vi "ActionVIOnDelete.vi"(6 "All deleted Refs":T1[](array[typedef]) format="%.0x", 8 "error in (no error)":errorcluster, 11 "Item Ref in":T1 format="%.0x") -> (0 "error out":errorcluster, 3 "Item Ref out":T1 format="%.0x")   [LabVIEW 2013, in "J1939 Addon System Explorer.lvlib"]
uses:
  J1939 Addon System Explorer.lvlib
  <vilib>/NI Veristand/Custom Device API/Custom Device Item Ref.ctl
  Shared/Types/XNET Settings.ctl
  Shared/SubVIs/Constants.vi
  <vilib>/NI Veristand/Custom Device API/Get Item Property (Variant).vi
  <vilib>/NI Veristand/Custom Device Tools/Custom Device Utility Library/NI VeriStand - Search for Item by GUID.vi
  <vilib>/NI Veristand/Custom Device Tools/Custom Device Utility Library/NI VeriStand - Search for Item by Name.vi
  Shared/J1939 Addon Shared.lvlib
  <vilib>/NI Veristand/Custom Device API/Custom Device API.lvlib
  <vilib>/NI Veristand/Custom Device Tools/Custom Device Utility Library/Custom Device Utility Library.lvlib
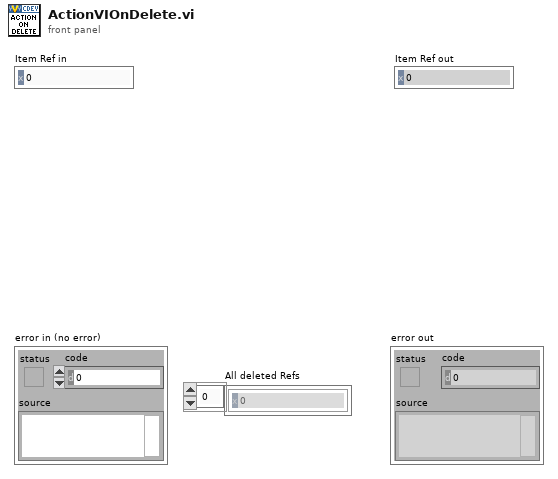
[diagram p1: front panel]
types:
  T1 = typedef "Custom Device API.lvlib/Custom Device Item Ref.ctl" = u64
  T2 = typedef "J1939 Addon Shared.lvlib/XNET Settings.ctl" = cluster{"Database":refnum<k21>, "Cluster":refnum<k21>, "Port":string, "Baud rate [Bd]":u32, "Termination":u32, "Incoming Rate":u32, "Outcoming Rate":u32, "Write Decimation":u32}
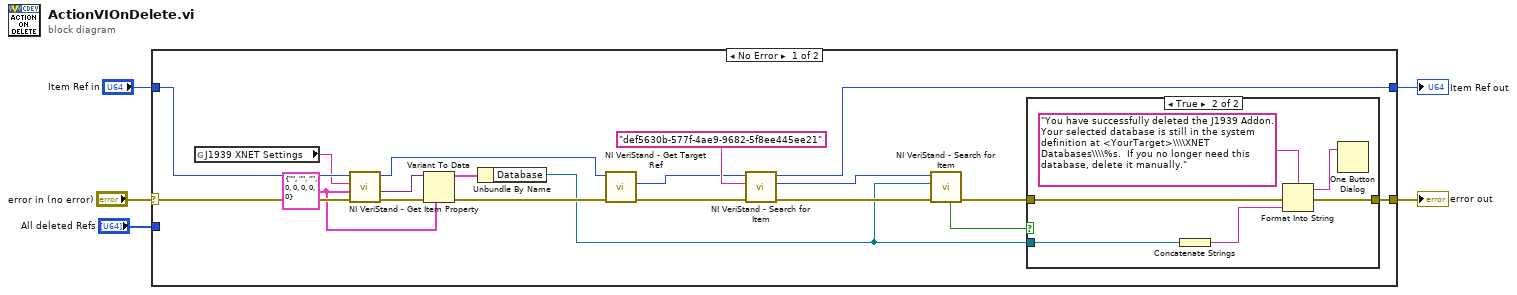
[diagram p0: block diagram]
diagram:
  n1 = case shown="No Error" "error in (no error)" {
    selector: "error in (no error)" -> [w24 w33]
    tunnel: [w22 w33] -> w4
    tunnel: "Item Ref in" -> [w23 w32]
    tunnel: [w21 w32] -> w2
    tunnel: "All deleted Refs" -> [_ _]
    frame No Error {
      w17 = T2 {"Database"="", "Cluster"="", "Port"="", "Baud rate [Bd]"=0, "Termination"=0, "Incoming Rate"=0, "Outcoming Rate"=0, "Write Decimation"=0} ("J1939 XNET Settings")
      n2 = global read "Constants.vi" "J1939 XNET Settings"() -> (w20:string)
      n3 = call-poly <vilib>:"NI VeriStand - Get Item Property.vi"("error in (no error)"=w24, "Default Value"=w17, "Property Name"=w20, "Item Ref in"=w23) -> ("error out"=w18:errorcluster, "Value"=w19:variant, "Item Ref out"=w10:T1)  [unwired: 4 in, 1 out]
      n4 = Variant To Data(error in=w18, type=w17, Variant=w19) -> (data=w16:T2, error out=w8:errorcluster)
      n5 = Unbundle By Name(w16) -> ("Database"=w6:refnum<k21>)
      n6 = call <vilib>:"NI VeriStand - Get Target Ref.vi"("error in"=w8, "Item Ref in"=w10) -> ("error out"=w7:errorcluster, "Target Ref"=w9:T1)  [unwired: 6 in, 2 out]
      n7 = call-poly <vilib>:"NI VeriStand - Search for Item.vi"("error in"=w7, "Item GUID"="def5630b-577f-4ae9-9682-5f8ee445ee21" ("string"), "Section Ref in"=w9) -> ("error out"=w13:errorcluster, "Item Ref"=w14:T1, "Section Ref out"=w21:T1)  [unwired: 5 in, 1 out]
      n8 = call-poly <vilib>:"NI VeriStand - Search for Item.vi"("error in"=w13, "Item Name"=w6, "Section Ref in"=w14) -> ("error out"=w12:errorcluster, "Found"=w11:bool)  [unwired: 5 in, 2 out]
      n9 = case shown="True" w11 {
        tunnel: w12 -> [w25 w31]
        tunnel: [w25 w30] -> w22
        tunnel: w6 -> [_ w27]
        frame False {
        }
        frame True {
          n10 = Concatenate Strings(w27) -> (w26:string)
          n11 = Format Into String(format string="You have successfully deleted the J1939 Addon.  Your selected database is still in the system definition at <YourTarget>\\\\XNET Databases\\\\%s.  If you no longer need this database, delete it manually." ("message"), error in=w31, w26) -> (resulting string=w28:string, error out=w30:errorcluster)  [unwired: 1 in]
          n12 = One Button Dialog(message=w28) -> ()  [unwired: 1 in, 1 out]
        }
      }
    }
    frame Error {
    }
  }
  "error out" <- w4
  "Item Ref out" <- w2
